vi "Convert to U32 array.vi"(9 "input valid":bool, 11 "data in":T1[](array[typedef])=[{"I"=0.0, "Q"=0.0, "overflow"=FALSE}, {"I"=0.0, "Q"=0.0, "overflow"=FALSE}, {"I"=0.0, "Q"=0.0, "overflow"=FALSE}, {"I"=0.0, "Q"=0.0, "overflow"=FALSE}, {"I"=0.0, "Q"=0.0, "overflow"=FALSE}, {"I"=0.0, "Q"=0.0, "overflow"=FALSE}, {"I"=0.0, "Q"=0.0, "overflow"=FALSE}, {"I"=0.0, "Q"=0.0, "overflow"=FALSE}]) -> (1 "output valid":bool, 2 "Array":u32[](array[numeric]), 3 "overflow":bool)   [LabVIEW 2015, in "DDC_7976R_v1.lvlib"]
uses:
  DDC_7976R_v1.lvlib
  <instrlib>/_niInstr/DSP/v1/Shared/Public/IQ Data.ctl
  <instrlib>/_niInstr/DSP/v1/Shared/niInstr DSP v1 Shared.lvlib
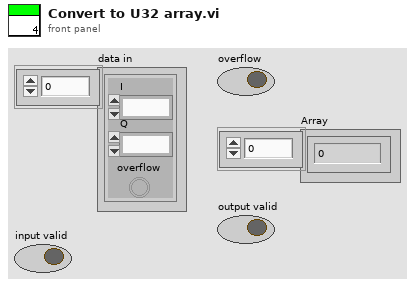
[diagram p1: front panel]
types:
  T1 = typedef "niInstr DSP v1 Shared.lvlib/IQ Data.ctl" = cluster{"I":fxp<+/-,18,1>, "Q":fxp<+/-,18,1>, "overflow":bool}
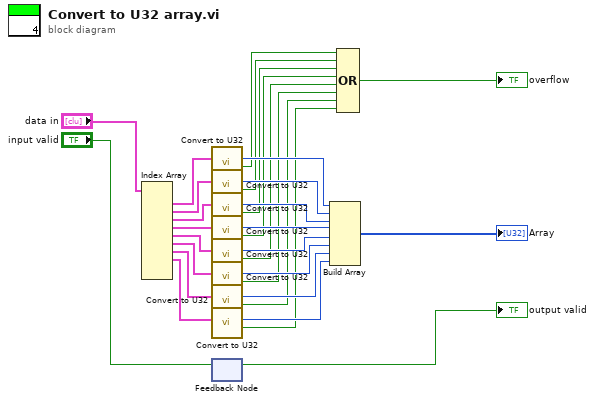
[diagram p0: block diagram]
diagram:
  n1 = Index Array(array="data in") -> (element #1=w21:T1, element #2=w20:T1, element #3=w19:T1, element #4=w18:T1, element #5=w17:T1, element #6=w16:T1, element #7=w15:T1, element #8=w14:T1)  [unwired: 10 in, 2 out]
  n2 = call "Convert to U32.vi"("data"=w21) -> ("overflow"=w1:bool, "Numeric Control"=w29:u32)  [unwired: 9 in]
  n3 = call "Convert to U32.vi"("data"=w20) -> ("overflow"=w2:bool, "Numeric Control"=w28:u32)  [unwired: 9 in]
  n4 = call "Convert to U32.vi"("data"=w19) -> ("overflow"=w3:bool, "Numeric Control"=w27:u32)  [unwired: 9 in]
  n5 = call "Convert to U32.vi"("data"=w18) -> ("overflow"=w5:bool, "Numeric Control"=w26:u32)  [unwired: 9 in]
  n6 = call "Convert to U32.vi"("data"=w17) -> ("overflow"=w6:bool, "Numeric Control"=w25:u32)  [unwired: 9 in]
  n7 = call "Convert to U32.vi"("data"=w16) -> ("overflow"=w7:bool, "Numeric Control"=w24:u32)  [unwired: 9 in]
  n8 = call "Convert to U32.vi"("data"=w15) -> ("overflow"=w8:bool, "Numeric Control"=w23:u32)  [unwired: 9 in]
  n9 = call "Convert to U32.vi"("data"=w14) -> ("overflow"=w9:bool, "Numeric Control"=w22:u32)  [unwired: 9 in]
  n10 = feedback #1() -> (→"output valid":bool)  [unwired: 1 in]
  n11 = feedback-in #1("input valid") -> ()
  n12 = Build Array(w29, w28, w27, w26, w25, w24, w23, w22) -> (→"Array":u32[])
  n13 = Compound Arithmetic op=OR(w1, w2, w3, w5, w6, w7, w8, w9) -> (→"overflow":bool)
